vi "SquareCont.vi"(9 "ContPow":T6, 11 "RectHatch":T1={"Width"=1.0, "Height"=2.0, "Angle"=45.0, "OffX"=0.1, "OffY"=0.1, "Spacing"=0.1} {"Spacing" format="%#_13g"; "OffY" format="%#_13g"; "OffX" format="%#_13g"; "Height" format="%#_13g"; "Width" format="%#_13g"}) -> (3 "PathSupreme":T2)   [LabVIEW 2014]
uses:
  TypeDefs/PowerSpeed.ctl
  TypeDefs/PathSupreme.ctl
  PSup2SCAN/Sub/VelocityProfile.ctl
  PSup2SCAN/Sub/PathCut.ctl
  PSup2SCAN/Sub/Segment.ctl
  TypeDefs/RectHatch.ctl
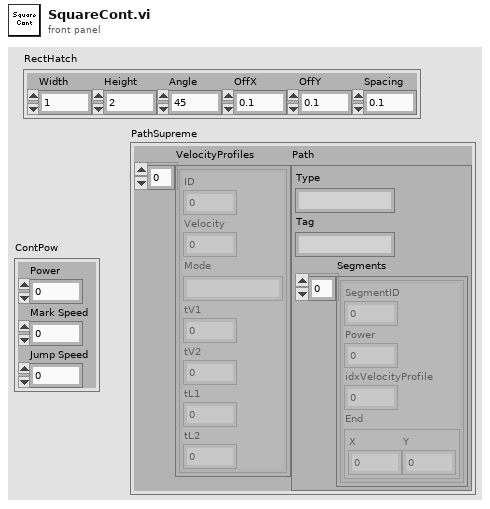
[diagram p1: front panel]
types:
  T1 = typedef "RectHatch.ctl" = cluster{"Width":dbl, "Height":dbl, "Angle":sgl, "OffX":dbl, "OffY":dbl, "Spacing":dbl}
  T2 = typedef "PathSupreme.ctl" = cluster{"VelocityProfiles":T3[], "Path":T4}
  T3 = typedef "VelocityProfile.ctl" = cluster{"ID":u32, "Velocity":dbl, "Mode":string, "tV1":u32, "tV2":u32, "tL1":u32, "tL2":u32}
  T4 = typedef "PathCut.ctl" = cluster{"Type":string, "Tag":string, "Segments":T5[]}
  T5 = typedef "Segment.ctl" = cluster{"SegmentID":u16, "Power":sgl, "idxVelocityProfile":u16, "End":cluster{"X":sgl, "Y":sgl}}
  T6 = typedef "PowerSpeed.ctl" = cluster{"Power":dbl, "Mark Speed":dbl, "Jump Speed":dbl}
  T7 = typedef "Point2DwSlope.ctl" = cluster{"X":sgl, "Y":sgl, "Slope":dbl}
  T8 = cluster{"VertexArray":T7[], "OnOffAr":enum16{"On", "Off"}[]}
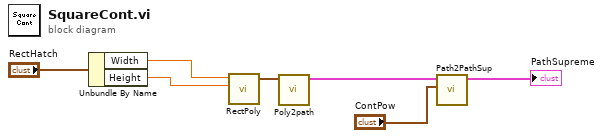
[diagram p0: block diagram]
diagram:
  n1 = Unbundle By Name("RectHatch") -> ("Width"=w2:dbl, "Height"=w1:dbl)
  n2 = call "RectPoly.vi"("Height"=w1, "Width"=w2) -> ("VertexArray"=w4:T7[])  [unwired: 9 in]
  n3 = call "Poly2path.vi"("VertexArray"=w4) -> ("Path"=w5:T8)  [unwired: 10 in]
  n4 = call "Path2PathSup.vi"("PowerSpeed"="ContPow", "Combined"=w5) -> ("PathSupreme"=→"PathSupreme":T2)  [unwired: 9 in]
